vi "ConvertCSVListToStringArray.vi"(11 "CSV List":string) -> (3 "String Array":string[](array[string]))   [LabVIEW 2012]
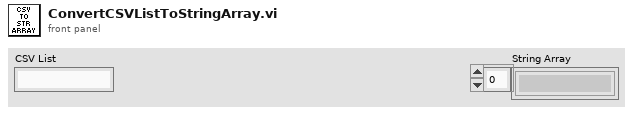
[diagram p1: front panel]
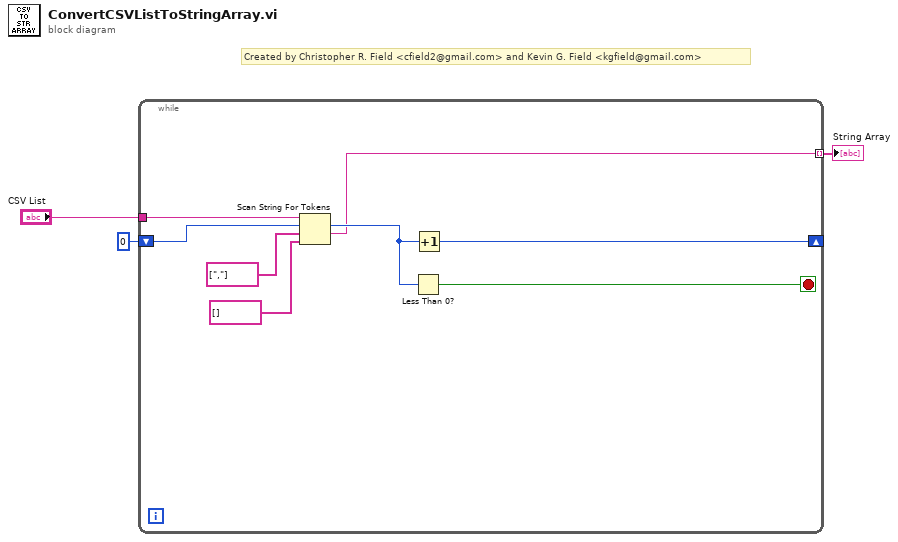
[diagram p0: block diagram]
diagram:
  # "Created by Christopher R. Field <cfield2@gmail.com> and Kevin G. Field <kgfield@gmail.com>"
  n1 = while {
    tunnel: "CSV List" -> [w11]
    shift-right: [w8] -> _
    shift-left: 0 -> [w7]
    tunnel: [w4] -> w1 mode=indexing
    stop <- w6 stop-if-true
    n2 = Scan String For Tokens(6:string[] [] ("delimiters (\\s,\\t,\\r,\\n)"), 7:string[] [","] ("operators (none)"), 8:w7, 9:w11) -> (1:w4:string, 2:w5:i32)  [unwired: 2 in, 2 out]
    n3 = Less Than 0?(x=w5) -> (x < 0?=w6:bool)
    n4 = Increment(x=w5) -> (x+1=w8:i32)
  }
  "String Array" <- w1
